vi "CNR_ConvertImageTo1DArray(Background).vi"(8 "error in (no error)":errorcluster, 11 "Refnum in":T1) -> (0 "error out":errorcluster, 3 "Array":dbl[](array[numeric]))   [LabVIEW 2023]
uses:
  <vilib>/vision/Image Controls.llb/IMAQ Image.ctl
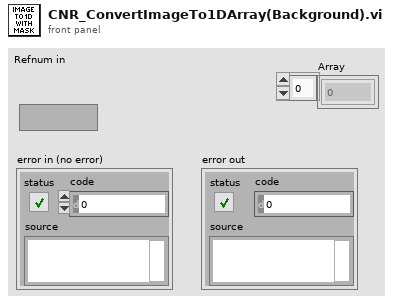
[diagram p1: front panel]
types:
  T1 = typedef "IMAQ Image.ctl" = refnum<image>
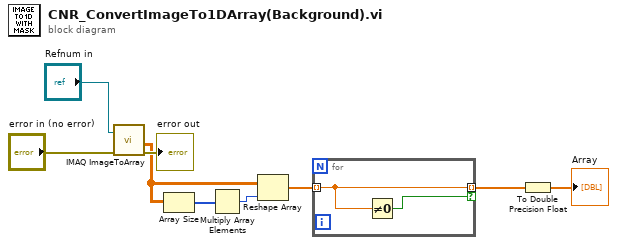
[diagram p0: block diagram]
diagram:
  n1 = call "IMAQ ImageToArray"("error in (no error)"="error in (no error)", "Image"="Refnum in") -> ("Image Pixels (Float)"=w3:sgl[][], "error out"=→"error out":errorcluster)  [unwired: 2 in, 3 out]
  n2 = Array Size(array=w3) -> (size(s)=w7:i32[])
  n3 = Multiply Array Elements(1:w7) -> (0:w5:i32)
  n4 = Reshape Array(w3, w5) -> (w4:sgl[])
  n5 = for {
    tunnel: w4 -> [w11] mode=indexing
    tunnel: [w11] -> w2 mode=indexing if=w10
    n6 = Not Equal To 0?(x=w11) -> (x != 0?=w10:bool)
  }
  n7 = To Double Precision Float(number=w2) -> (double precision float=→"Array":dbl[])
